vi "references.vi"(7 "String in in":string, 11 "String in 3":string) -> (3 "String out":string)   [LabVIEW 2017]
uses:
  <userlib>/_NEVSTOP/Communicable State Machine(CSM)/Communicable State Machine.lvlib
  INI-Static-Variable-Support/INI-Static-Variable-Support.lvlib
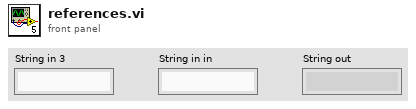
[diagram p1: front panel]
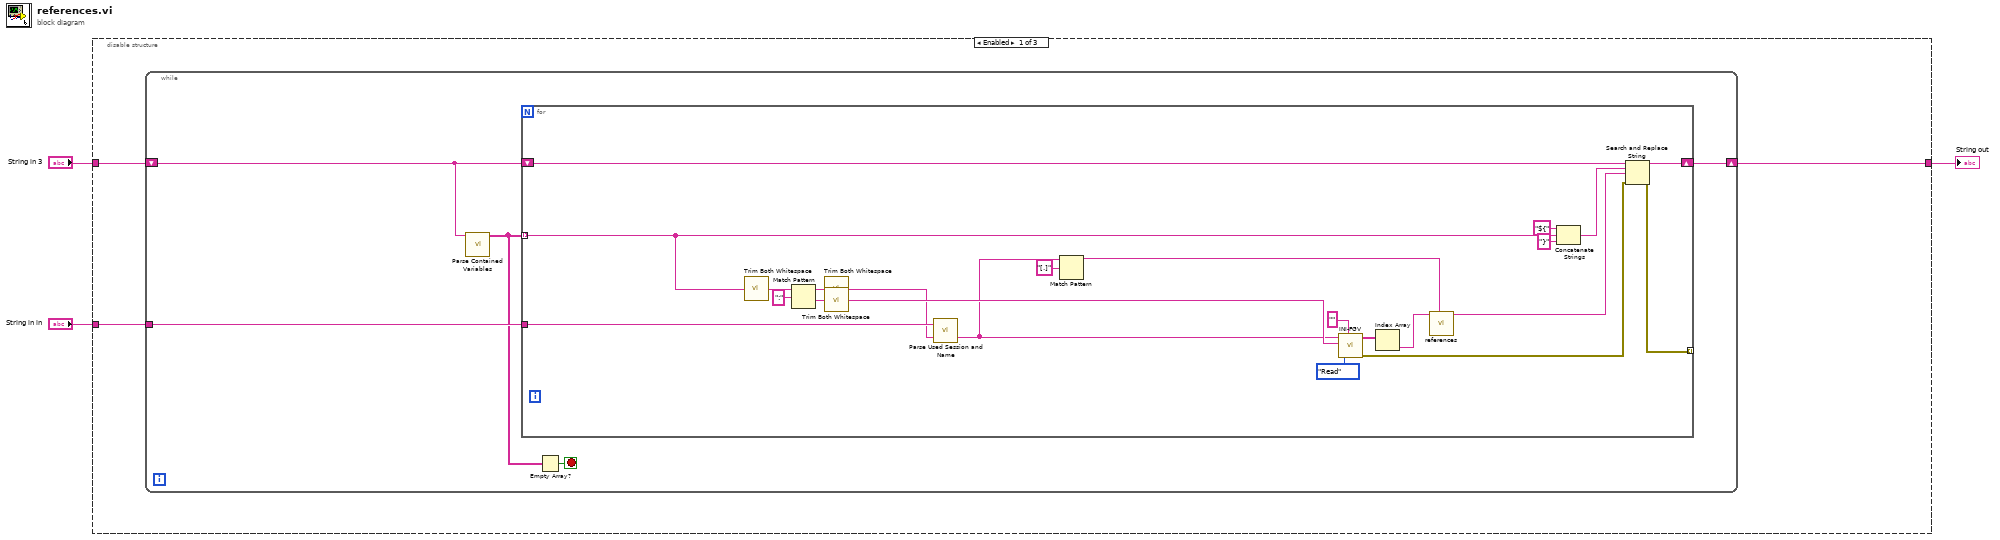
[diagram p0: block diagram]
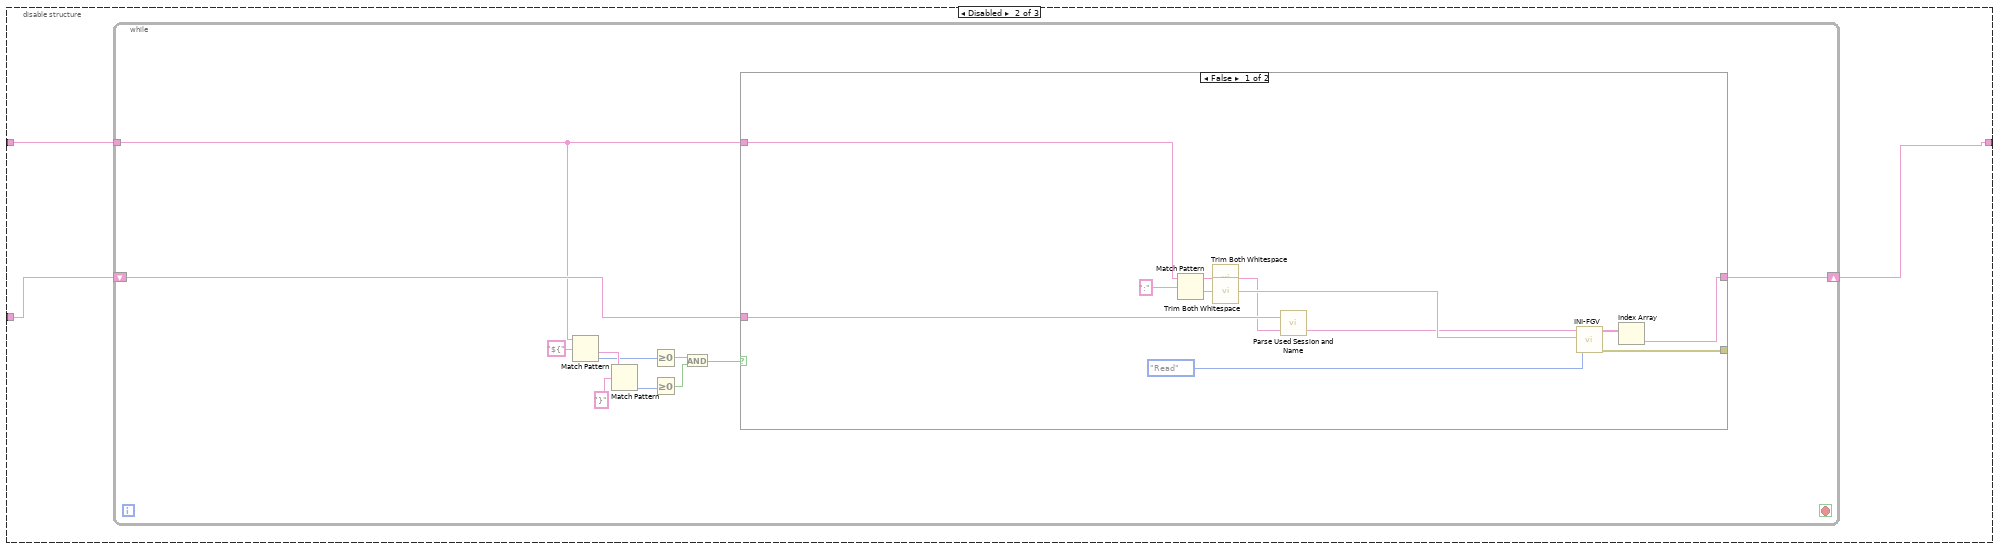
[diagram p2: hidden frame]
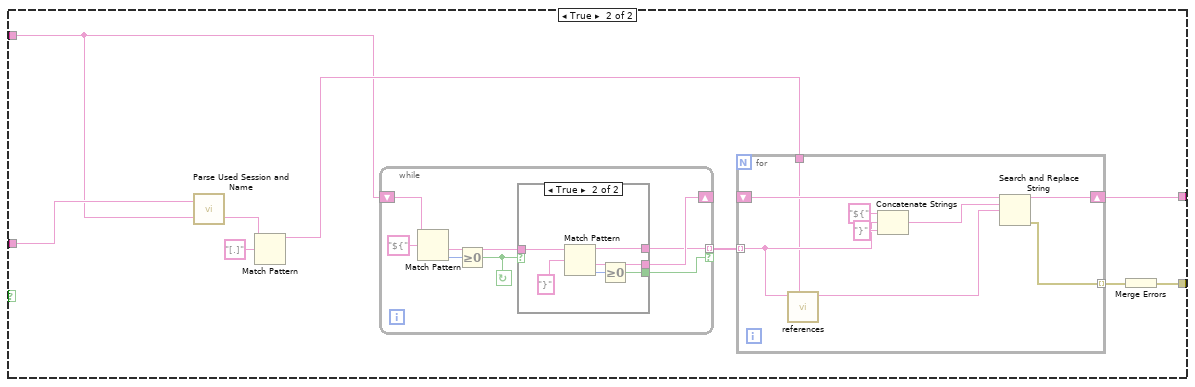
[diagram p3: hidden frame]
diagram:
  n1 = disable-structure shown="Enabled" {
    disable-tunnel: [w6 w35 _] -> w3
    disable-tunnel: "String in in" -> [w5 w37 _]
    disable-tunnel: "String in 3" -> [w4 w36 _]
    frame Enabled {
      n2 = while {
        shift-right: [w10] -> w6
        shift-left: w4 -> [w8]
        tunnel: w5 -> [w11]
        stop <- w9 stop-if-true
        n3 = call "Parse Contained Variables.vi"("String"=w8) -> ("Contained Variables"=w7:string[])  [unwired: 10 in]
        n4 = for {
          tunnel: w7 -> [w26] mode=indexing
          shift-right: [w31] -> w10
          shift-left: w8 -> [w32]
          tunnel: [w29] -> _ mode=indexing
          tunnel: w11 -> [w27]
          n5 = call <userlib>:"Trim Both Whitespace.vi"("String"=w26) -> ("Trimmed String"=w16:string)  [unwired: 1 in]
          n6 = Match Pattern(string=w16, regular expression=":") -> (before substring=w24:string, after substring=w23:string)  [unwired: 1 in, 2 out]
          n7 = call <userlib>:"Trim Both Whitespace.vi"("String"=w24) -> ("Trimmed String"=w21:string)  [unwired: 1 in]
          n8 = call <userlib>:"Trim Both Whitespace.vi"("String"=w23) -> ("Trimmed String"=w22:string)  [unwired: 1 in]
          n9 = call "Parse Used Session and Name.vi"("name"=w21, "Section Name(\"\" as Default)"=w27) -> ("used name"=w20:string)  [unwired: 1 in]
          n10 = Match Pattern(string=w20, regular expression="[.]") -> (before substring=w15:string)  [unwired: 1 in, 3 out]
          n11 = call "INI-FGV.vi"("Enum"=enum16{"Read", "Write", "Sync"}."Read", "Prefered Section"="", ">> Default Value >>"=w22, ">> Variable Name >>"=w20) -> ("error out"=w28:errorcluster, "Array"=w18:string[])  [unwired: 4 in, 2 out]
          n12 = Index Array(array=w18) -> (element=w14:string)  [unwired: 1 in]
          n13 = call "references.vi"("String in in"=w15, "String in 3"=w14) -> ("String out"=w13:string)  [unwired: 9 in]
          n14 = Concatenate Strings("${" ("regular expression"), w26, "}" ("regular expression")) -> (w30:string)
          n15 = Search and Replace String(input string=w32, search string=w30, replace string=w13, error in=w28) -> (result string=w31:string, error out=w29:errorcluster)  [unwired: 4 in, 2 out]
        }
        n16 = Empty Array?(array=w7) -> (empty?=w9:bool)
      }
    }
    frame Disabled {
      n17 = while {
        tunnel: w36 -> [w39]
        shift-right: [w38] -> w35
        shift-left: w37 -> [w48]
        stop <- _ stop-if-true
        n18 = Match Pattern(string=w39, regular expression="${") -> (after substring=w45:string, offset past match=w44:i32)  [unwired: 1 in, 2 out]
        n19 = Match Pattern(string=w45, regular expression="}") -> (offset past match=w43:i32)  [unwired: 1 in, 3 out]
        n20 = Greater Or Equal To 0?(x=w44) -> (x >= 0?=w42:bool)
        n21 = Greater Or Equal To 0?(x=w43) -> (x >= 0?=w41:bool)
        n22 = And(x=w42, y=w41) -> (x .and. y?=w40:bool)
        n23 = case shown="False" w40 {
          tunnel: [w50 w62] -> _
          tunnel: w48 -> [w54 w64]
          tunnel: [w51 w67] -> w38
          tunnel: w39 -> [w49 w61]
          frame False {
            n24 = Match Pattern(string=w49, regular expression=":") -> (before substring=w59:string, after substring=w58:string)  [unwired: 1 in, 2 out]
            n25 = call <userlib>:"Trim Both Whitespace.vi"("String"=w59) -> ("Trimmed String"=w53:string)  [unwired: 1 in]
            n26 = call <userlib>:"Trim Both Whitespace.vi"("String"=w58) -> ("Trimmed String"=w55:string)  [unwired: 1 in]
            n27 = call "Parse Used Session and Name.vi"("name"=w53, "Section Name(\"\" as Default)"=w54) -> ("used name"=w52:string)  [unwired: 1 in]
            n28 = call "INI-FGV.vi"("Enum"=enum16{"Read", "Write", "Sync"}."Read", ">> Default Value >>"=w55, ">> Variable Name >>"=w52) -> ("error out"=w50:errorcluster, "Array"=w57:string[])  [unwired: 5 in, 2 out]
            n29 = Index Array(array=w57) -> (element=w51:string)  [unwired: 1 in]
          }
          frame True {
            n30 = call "Parse Used Session and Name.vi"("name"=w61, "Section Name(\"\" as Default)"=w64) -> ("used name"=w65:string)  [unwired: 1 in]
            n31 = Match Pattern(string=w65, regular expression="[.]") -> (before substring=w63:string)  [unwired: 1 in, 3 out]
            n32 = while {
              shift-right: [w83] -> _
              shift-left: w61 -> [w84]
              tunnel: [w80] -> w69 mode=indexing if=w79
              stop <- w81 continue-if-true
              n33 = Match Pattern(string=w84, regular expression="${") -> (after substring=w85:string, offset past match=w82:i32)  [unwired: 1 in, 2 out]
              n34 = Greater Or Equal To 0?(x=w82) -> (x >= 0?=w81:bool)
              n35 = case shown="True" w81 {
                tunnel: w85 -> [w87 w93]
                tunnel: [w87 w92] -> w83
                tunnel: [_ w90] -> w80
                tunnel: [_ w88] -> w79
                frame False {
                }
                frame True {
                  n36 = Match Pattern(string=w93, regular expression="}") -> (before substring=w90:string, after substring=w92:string, offset past match=w89:i32)  [unwired: 1 in, 1 out]
                  n37 = Greater Or Equal To 0?(x=w89) -> (x >= 0?=w88:bool)
                }
              }
            }
            n38 = for {
              tunnel: w69 -> [w74] mode=indexing
              tunnel: [w72] -> w68 mode=indexing
              shift-right: [w71] -> w67
              shift-left: _ -> [w75]
              tunnel: w63 -> [w70]
              n39 = call "references.vi"("String in in"=w70, "String in 3"=w74) -> ("String out"=w73:string)  [unwired: 9 in]
              n40 = Concatenate Strings("${" ("regular expression"), w74, "}" ("regular expression")) -> (w78:string)
              n41 = Search and Replace String(input string=w75, search string=w78, replace string=w73) -> (result string=w71:string, error out=w72:errorcluster)  [unwired: 5 in, 2 out]
            }
            n42 = Merge Errors(w68) -> (w62:errorcluster)
          }
        }
      }
    }
    frame Disabled {
    }
  }
  "String out" <- w3
